vi "运维调试_氨氮.vi"() -> ()   [LabVIEW 2016, in "斯坦道氨氮.lvlib"]
uses:
  <vilib>/Utility/miscctls.llb/LVPointTypeDef.ctl
  <vilib>/Utility/config.llb/NI_LVConfig.lvlib
  <vilib>/ptbypt/NI_PtbyPt.lvlib
panel:
  in  "定时设置":cluster{"启动":bool, "控制命令":T1}(xcontrol)
  out "二级权限":bool
  out "一级权限":bool
  out "输入密码":u32
  out "布尔":bool
  in  "仪器参数设置":bool
  in  "流程固件":bool
  in  "量程参数读取":T2
  in  "模块启用":bool
  in  "串口设置":bool
  in  "公式一键写入":bool
  in  "流程路径":path=path "C:/Users/STD/Documents/斯坦道流程文件/流程.xml"
  in  "曲线模型":cluster{"X^2":dbl, "X":dbl, "B":dbl}(xcontrol)
  out "字符串":string
  in  "质控参数设置":bool
  in  "自动测试量程配置":T3
  out "温度2":sgl
  out "温度1":sgl
  out "ADC":sgl
  out "固件版本号":string
  in  "数组":string[](array[string])
  in  "量程切换阈值写入":bool
  in  "量程切换阈值读取":bool
  in  "参数下拉列表":enum16{"总磷", "总氮", "氨氮"}(ring)=enum."氨氮"
  in  "量程下拉列表":enum16{"低量程", "高量程"}(ring)
  in  "测量模式下拉列表":enum16{"水样测量", "零点核查", "跨度核查", "标样核查", "加标回收"}(ring)
  in  "公式":cluster{"X^2":dbl, "X":dbl, "b":dbl}
  in  "写公式":bool
  in  "读公式":bool
  in  "返回":bool
  in  "设置":bool
  out "序列号":string="序列号"
  out "测量数据":T4(xcontrol)
  out "集成报警信息":string
  out "总磷总氮运行状态":T5(xcontrol)
  in  "停止":bool
  in  "手动启动":bool
  in  "单步测试":bool
  in  "总磷氨氮调试":u16[](xcontrol)
  out "F3":sgl format="%#.6f"
  out "F2":sgl format="%#.6f"
  out "F1":sgl format="%#.6f"
  out "F0":sgl format="%#.6f"
  out "多列列表框":i32(listbox)
  # "参数设置"
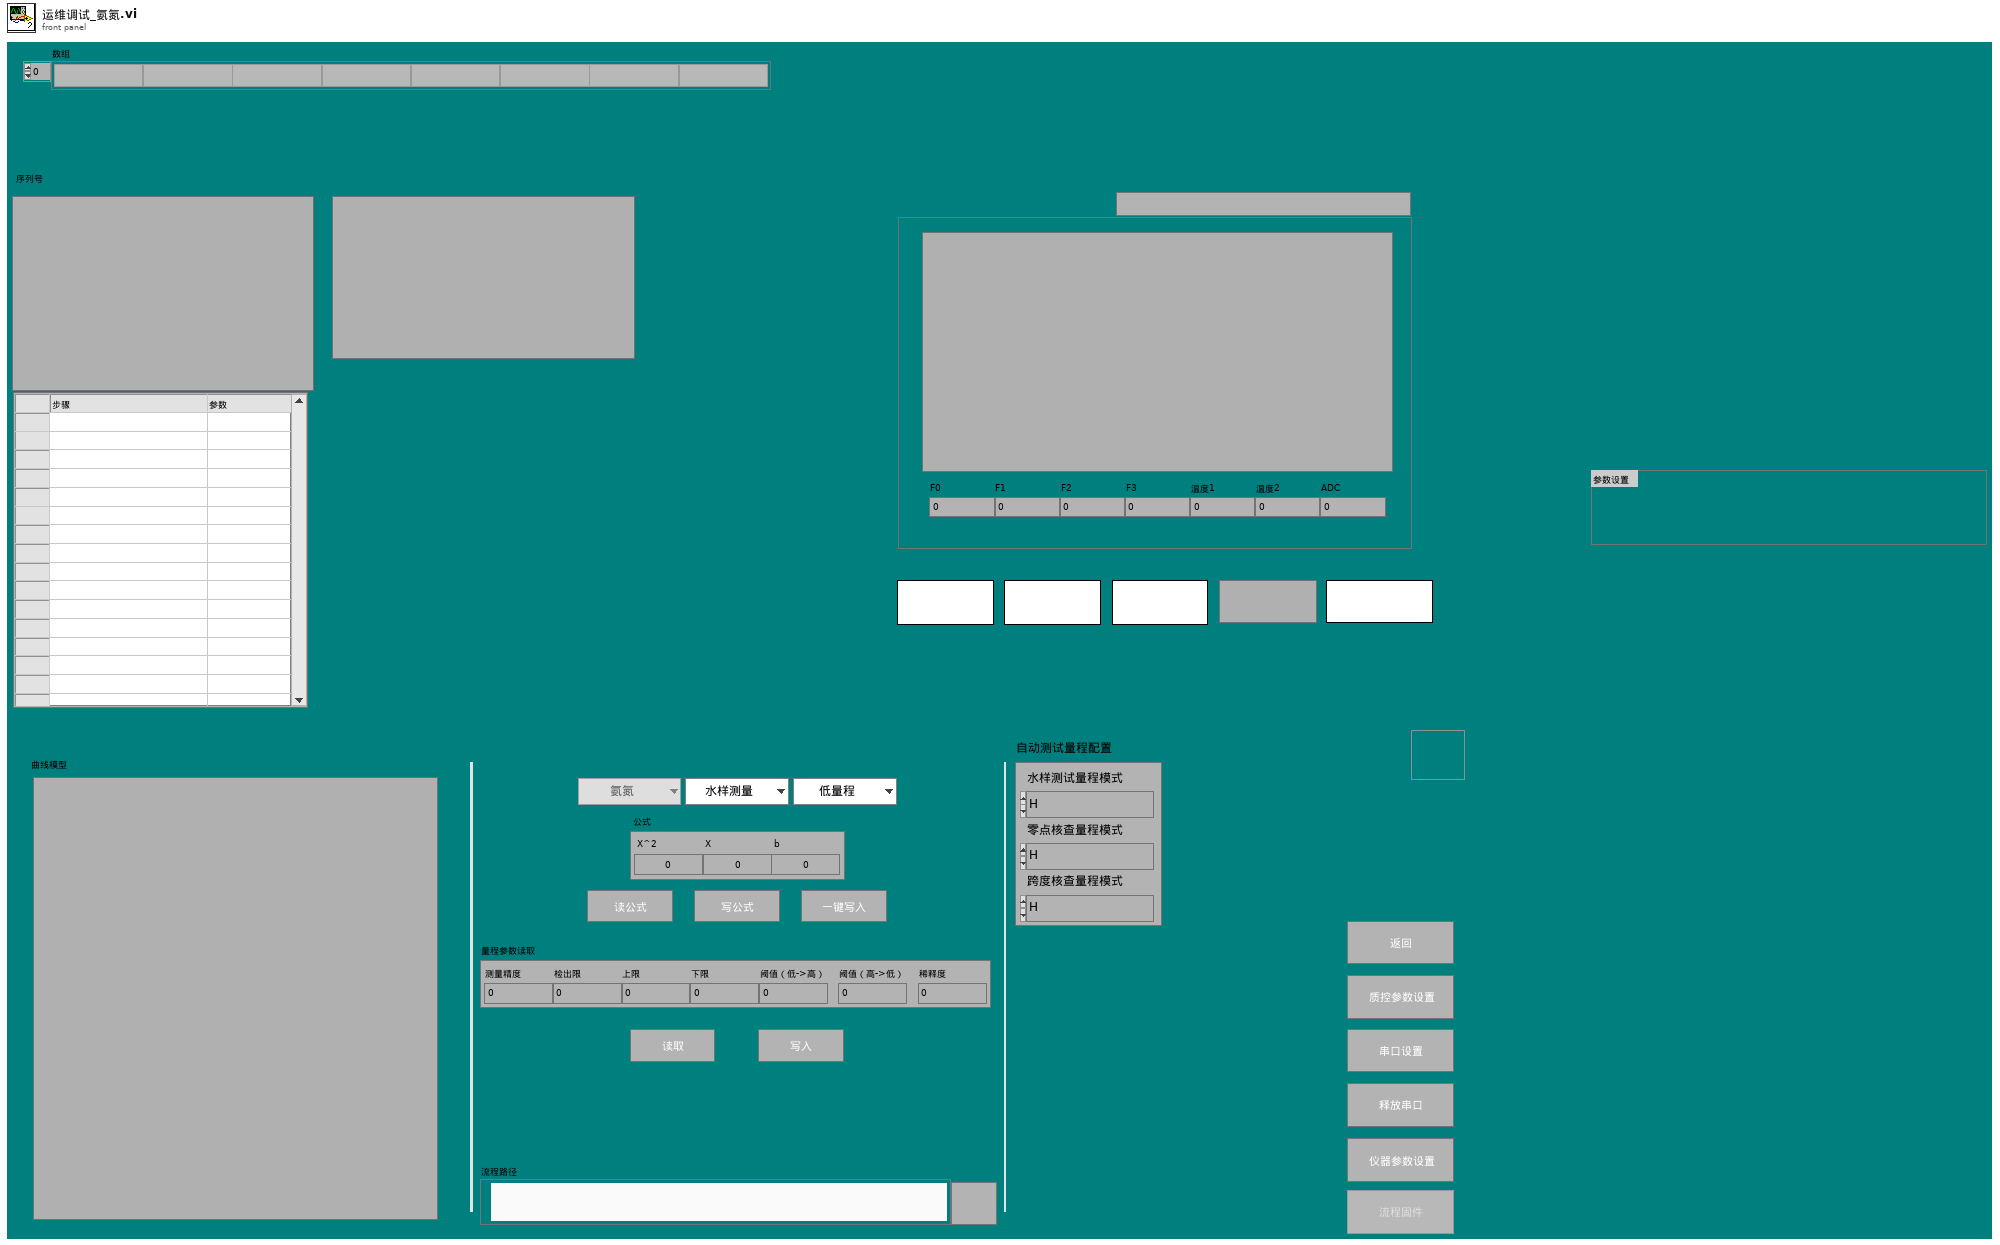
[diagram p1: front panel]
types:
  T1 = typedef "定时设置.xctl/国标控制命令.ctl" = enum16{"启动测量", "标样核查", "零点核查", "跨度核查", "空白测试", "平行样测试", "加标回收", "空白校准", "标样校准", "初始化（清洗）", "停止测试", "仪器重启", "校时", "模式设置", "测量间隔设置"}
  T2 = cluster{"测量精度":dbl, "检出限":dbl, "上限":dbl, "下限":dbl, "阈值（低->高）":dbl, "阈值（高->低）":dbl, "稀释度":dbl}
  T3 = cluster{"水样测试量程模式":enum16{"H", "L", "AUTO"}, "空白核查量程模式":enum16{"H", "L", "AUTO"}, "跨度核查量程模式":enum16{"H", "L", "AUTO"}}
  T4 = cluster{"flowid":u16, "测量精度":u16, "测量数据区":cluster{"因子编码":u32, "单位":u16, "标样参考值":sgl, "水样数据时间":timestamp, "水样实测值":sgl, "水样数据标识":string, "标样数据时间":timestamp, "标样实测值":sgl, "标样数据标识":string, "空白数据时间":timestamp, "空白实测值":sgl, "空白数据标识":string, "零点核查数据时间":timestamp, "零点核查实测值":sgl, "零点核查数据标识":string, "跨度核查数据时间":timestamp, "跨度核查实测值":sgl, "跨度核查数据标识":string, "加标回收数据时间":timestamp, "加标回收实测值":sgl, "加标回收数据标识":string, "平行样数据时间":timestamp, "平行样实测值":sgl, "平行样数据标识":string, "F0":sgl, "F1":sgl, "F2":sgl, "F3":sgl, "F4":sgl, "F5":sgl, "F6":sgl, "F7":sgl, "温度":sgl, "湿度":sgl, "X值":sgl, "fidrange":sgl}}
  T5 = cluster{"系统时间":timestamp, "工作状态":enum16{"空闲", "水样测试", "标样核查", "零点核查", "跨度核查", "空白测试", "平行样测试", "加标回收", "空白校准", "标样校准", "初始化（清洗）"}, "测量模式":enum16{"待机", "连续模式", "周期模式", "定点模式", "受控模式", "手动模式"}, "告警代码":u16, "故障代码":u16, "日志代码":u16, "软件版本":u16, "F0":sgl, "F1":sgl, "F2":sgl, "F3":sgl, "T":sgl, "H":sgl, "id":u16, "flowid":u16, "量程":u16, "总磷控温温度1":sgl, "营养盐控温温度2":sgl, "ADC":sgl}
  T6 = typedef "NI_LVConfig.lvlib/Config Data RefNum.ctl" = refnum<k1>
  T7 = typedef "LVPointTypeDef.ctl" = cluster{"Horizontal":i16, "Vertical":i16}
  T8 = cluster{"因子编码":u32, "单位":u16, "标样参考值":sgl, "水样数据时间":timestamp, "水样实测值":sgl, "水样数据标识":string, "标样数据时间":timestamp, "标样实测值":sgl, "标样数据标识":string, "空白数据时间":timestamp, "空白实测值":sgl, "空白数据标识":string, "零点核查数据时间":timestamp, "零点核查实测值":sgl, "零点核查数据标识":string, "跨度核查数据时间":timestamp, "跨度核查实测值":sgl, "跨度核查数据标识":string, "加标回收数据时间":timestamp, "加标回收实测值":sgl, "加标回收数据标识":string, "平行样数据时间":timestamp, "平行样实测值":sgl, "平行样数据标识":string, "F0":sgl, "F1":sgl, "F2":sgl, "F3":sgl, "F4":sgl, "F5":sgl, "F6":sgl, "F7":sgl, "温度":sgl, "湿度":sgl, "X值":sgl, "fidrange":u16}
  T9 = enum16{"空闲", "水样测试", "标样核查", "零点核查", "跨度核查", "空白测试", "平行样测试", "加标回收", "空白校准", "标样校准", "初始化（清洗）"}
  T10 = enum32{"Bad", "Idle", "Run top level", "Running"}
  T11 = typedef "定时设置.xctl/周期模式设置.ctl" = enum16{"不启用", "定点模式", "间隔模式"}
  T12 = typedef "定时设置.xctl/定点周期设置.ctl" = cluster{"启动命令":T13, "启动命令 2":T13, "启动命令 3":T13, "启动命令 4":T13, "启动命令 5":T13, "启动命令 6":T13, "启动命令 7":T13, "启动命令 8":T13, "启动命令 9":T13, "启动命令 10":T13, "启动命令 11":T13, "启动命令 12":T13, "启动命令 13":T13, "启动命令 14":T13, "启动命令 15":T13, "启动命令 16":T13, "启动命令 17":T13, "启动命令 18":T13, "启动命令 19":T13, "启动命令 20":T13, "启动命令 21":T13, "启动命令 22":T13, "启动命令 23":T13, "启动命令 24":T13}
  T13 = typedef "定时设置.xctl/启动命令选择.ctl" = u16
  T14 = typedef "定时设置.xctl/间隔启动设置.ctl" = cluster{"启动命令":T13, "启动间隔":dbl, "启动次数":i32}
  T15 = enum8{"Enabled", "Disabled", "Disabled and Grayed Out"}
  T16 = cluster{"启动模式":enum16{"跨度核查", "水样测量", "空白核查", "标样核查", "加标回收"}, "启动参数":u16, "量程":enum16{"低量程", "高量程"}}
  T17 = cluster{"时间标识":timestamp, "设备":string, "日志信息":string, "流程参数":string}
  T18 = cluster{"时间标识":timestamp, "设备":string, "日志信息":string}
  T19 = typedef "LVRowAndColumnUnsignedTypeDef.ctl" = cluster{"Row":u32, "Column":u32}
  T20 = cluster{"参数下拉列表":enum16{"总磷", "总氮", "氨氮"}, "测量模式下拉列表":enum16{"水样测量", "零点核查", "跨度核查", "标样核查", "加标回收"}, "量程下拉列表":enum16{"低量程", "高量程"}}
  T21 = cluster{"站号":u16, "量程切换":enum32{"H", "L", "AUTO"}, "控制命令":enum16{"启动测量", "标样核查", "零点核查", "跨度核查", "空白测试", "平行样测试", "加标回收", "空白校准", "标样校准", "初始化（清洗）", "停止测试", "仪器重启", "校时", "模式设置", "测量间隔设置"}, "模式设置":enum16{"待机", "连续模式", "周期模式", "定点模式", "受控模式", "手动模式"}, "测量间隔":u16}
  T22 = cluster{"跨度值":dbl, "零点标准液浓度":dbl, "跨度标准液浓度":dbl, "标准液标准浓度":dbl}
  T23 = cluster{"确定":bool, "跨度值":dbl, "零点标准液浓度":dbl, "跨度标准液浓度":dbl, "标准液标准浓度":dbl}
  T24 = cluster{"测量量程":dbl, "测量精度":dbl, "测量间隔":dbl, "消解温度":dbl, "消解时长":dbl, "空白校准时间":timestamp, "曲线截距":dbl, "曲线斜率":dbl, "测量检出限":dbl, "测量信号值":dbl, "线性相关系数":dbl, "二次多项式系数":dbl, "标样校准时间":timestamp, "单位":u16}
  T25 = cluster{"确定":bool, "测量量程":dbl, "测量精度":dbl, "测量间隔":dbl, "消解温度":dbl, "消解时长":dbl, "空白校准时间":timestamp, "曲线截距":dbl, "曲线斜率":dbl, "测量检出限":dbl, "测量信号值":dbl, "线性相关系数":dbl, "二次多项式系数":dbl, "标样校准时间":timestamp, "单位":u16}
  T26 = cluster{"测量精度":u16, "检出限":dbl, "上限":dbl, "下限":dbl, "阈值（低->高）":dbl, "阈值（高->低）":dbl, "稀释度":dbl}
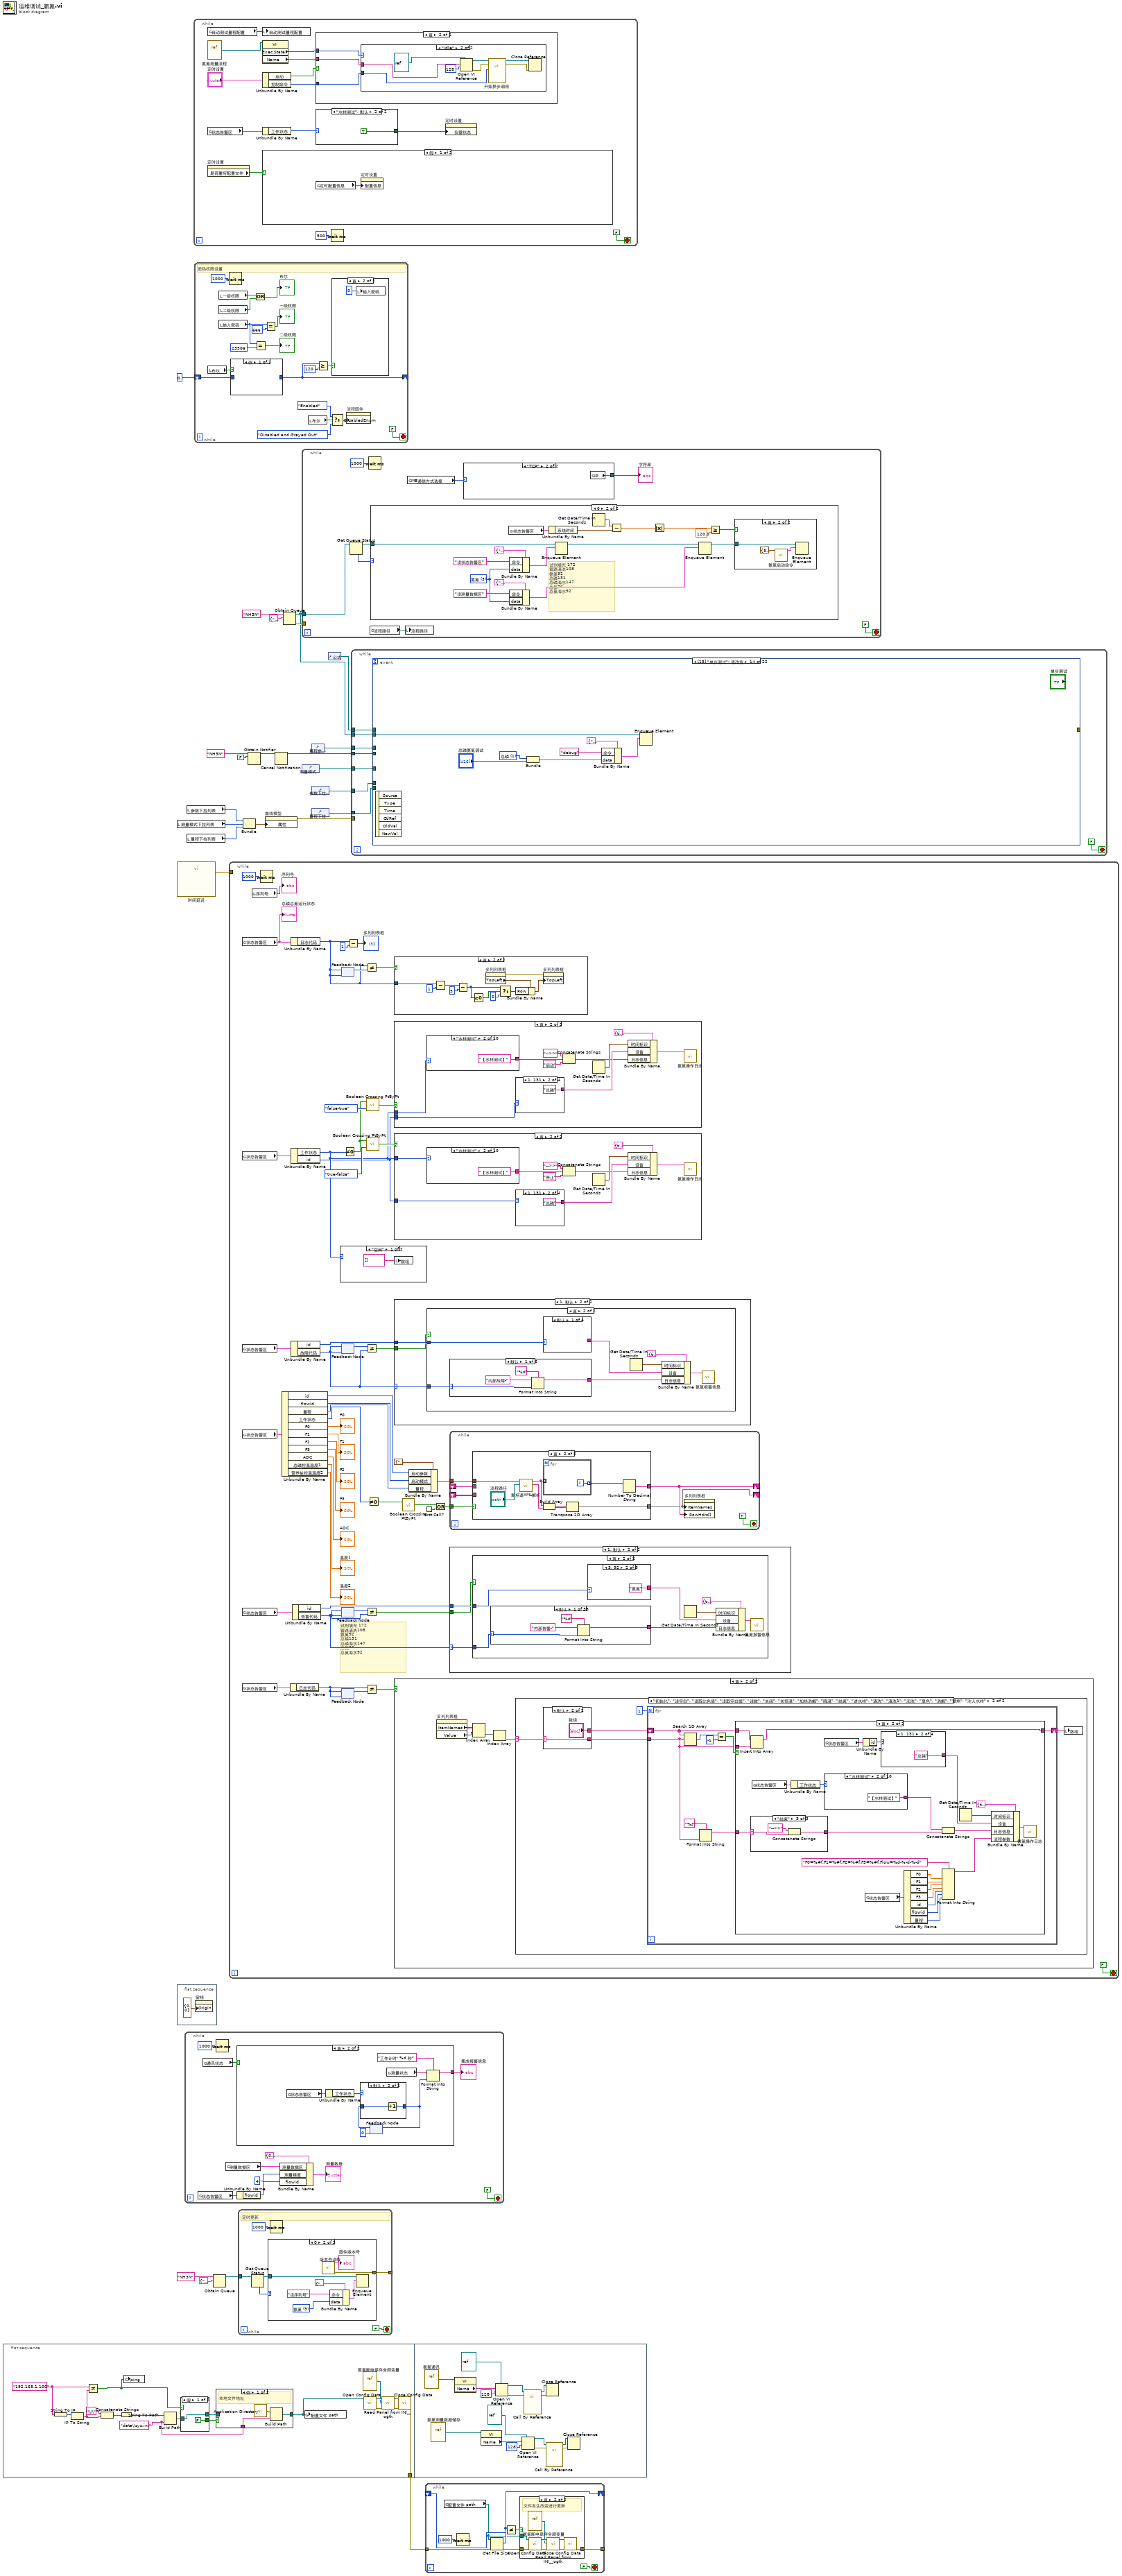
[diagram p0: block diagram]
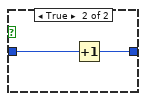
[diagram p4: hidden frame]
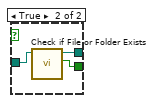
[diagram p5: hidden frame]
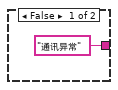
[diagram p8: hidden frame]
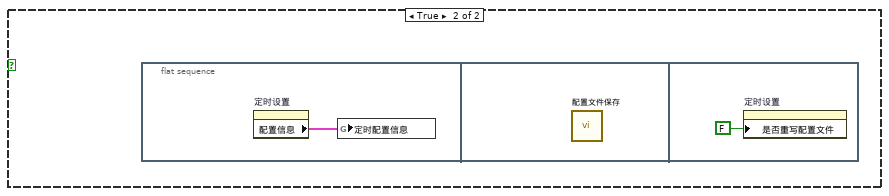
[diagram p10: hidden frame]
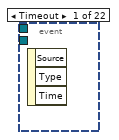
[diagram p14: hidden frame]
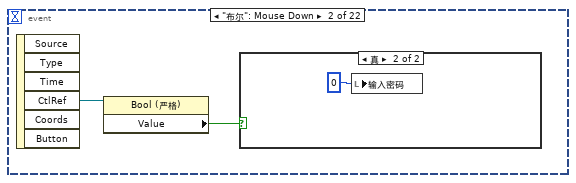
[diagram p15: hidden frame]
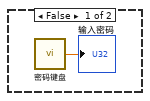
[diagram p16: hidden frame]
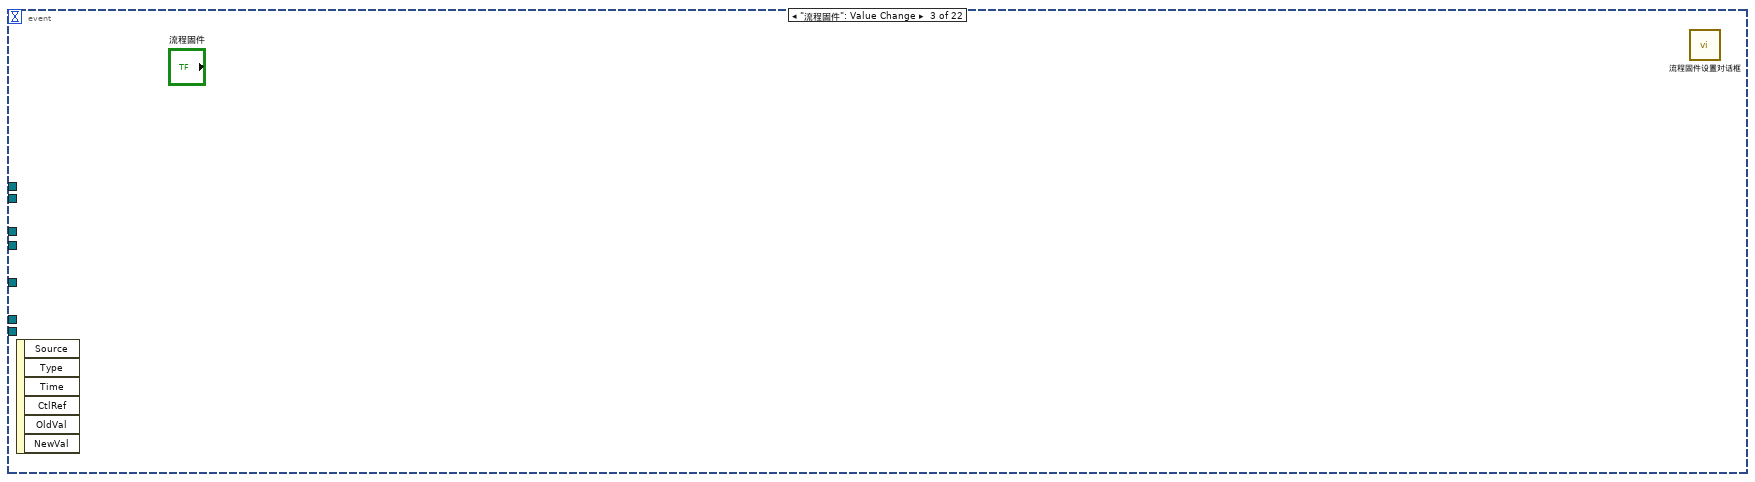
[diagram p17: hidden frame]
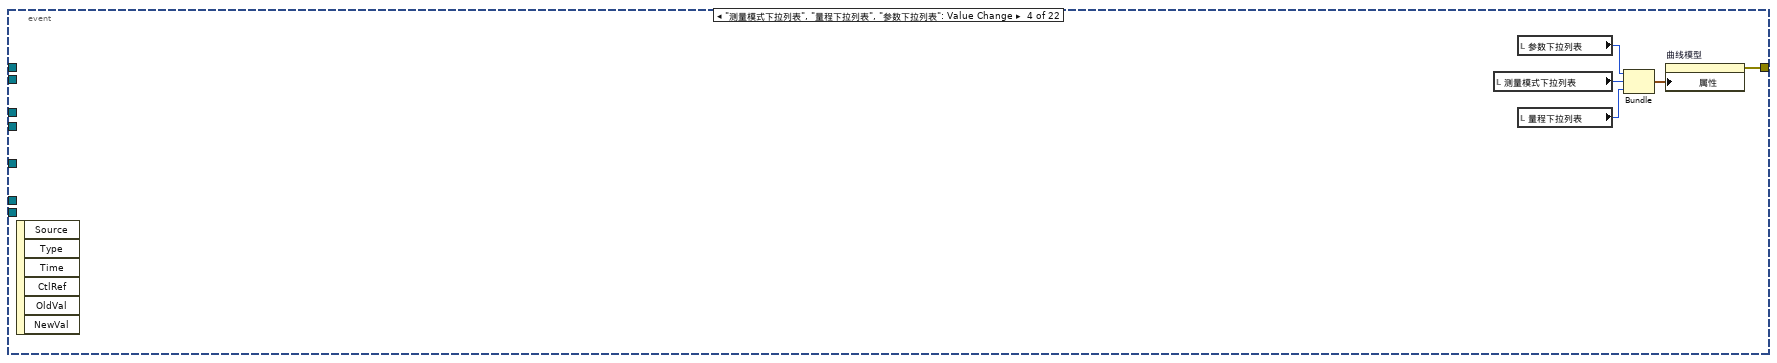
[diagram p18: hidden frame]
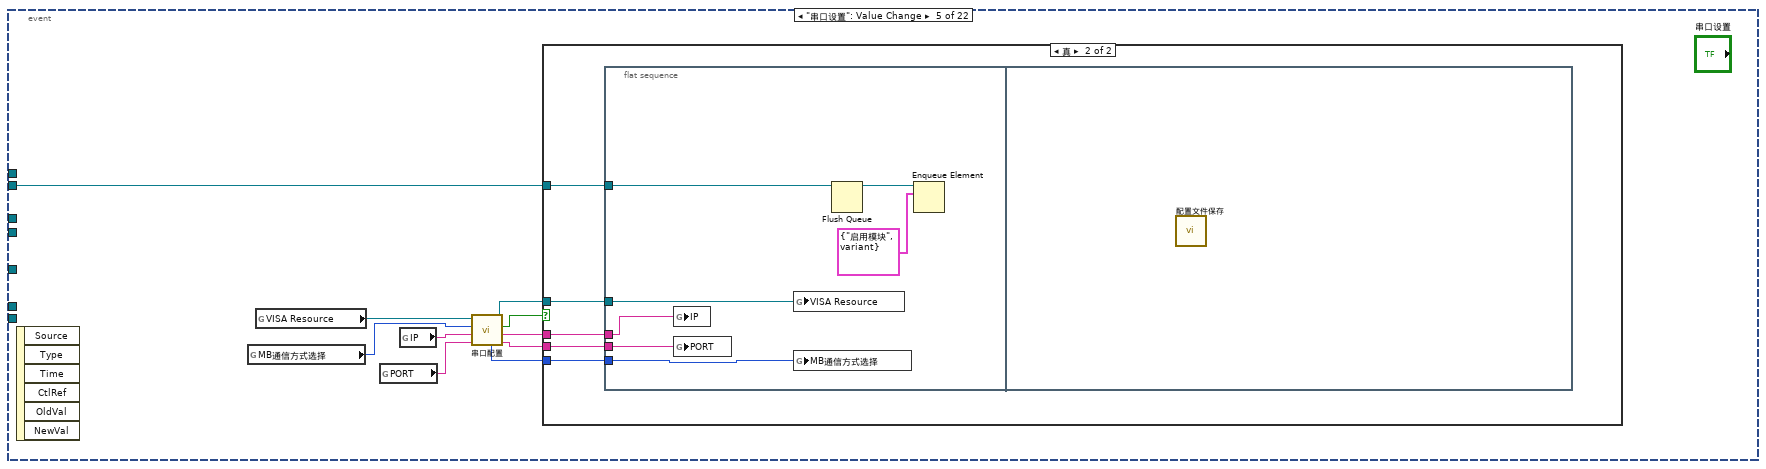
[diagram p19: hidden frame]
diagram:
  n1 = flat-sequence {
    tunnel: [w25] -> w1
    frame #0 {
      w36 = "data\\sys.ini" ("名称或相对路径")
      w28 = "192.168.1.100" ("名称")
      n2 = String To IP(1:w28) -> (0:w35:u32)
      n3 = IP To String(2:w35) -> (0:w32:string)  [unwired: 1 in]
      n4 = Not Equal?(x=w28, y=w32) -> (x != y?=w37:bool)
      n5 = Concatenate Strings("\\\\" ("字符串"), w32) -> (w33:string)
      n6 = String To Path(string=w33) -> (path=w27:path)
      n7 = global write "VAR氨氮全局变量.vi" "ping"(w37) -> ()
      n8 = Build Path(base path=w27, name or relative path=w36) -> (appended path=w31:path)
      n9 = case shown="假" w37 {
        tunnel: w31 -> [w43 w47]
        tunnel: [w43 w46] -> w30
        tunnel: [FALSE w45] -> w29
        frame False {
        }
        frame True {
          n10 = call <vilib>:"Check if File or Folder Exists.vi"("path"=w47) -> ("file or folder exists?"=w45:bool, "dup path"=w46:path)  [unwired: 8 in, 1 out]
        }
      }
      n11 = case shown="假" w29 {
        tunnel: w30 -> [_ w51]
        tunnel: [w49 w51] -> w26
        tunnel: w36 -> [w48 _]
        frame False {
          # "本地文件地址"
          n12 = call <vilib>:"Application Directory.vi"() -> ("Application Directory"=w50:path)
          n13 = Build Path(base path=w50, name or relative path=w48) -> (appended path=w49:path)
        }
        frame True {
          # "网络共享地址"
        }
      }
      n14 = global write "VAR氨氮全局变量.vi" "配置文件 path"(w26) -> ()
      n15 = vi-ref "氨氮断电保存全局变量.vi"() -> (w41:refnum<vi>)
      n16 = call <vilib>:"Open Config Data.vi"("configuration file path"=w26) -> ("error out"=w39:errorcluster, "refnum"=w42:T6)  [unwired: 8 in, 1 out]
      n17 = call <userlib>:"Read Panel from INI__ogtk.vi"("error in (no error)"=w39, "VI ref"=w41, "refnum"=w42) -> ("error out"=w38:errorcluster, "refnum out"=w40:T6)  [unwired: 7 in]
      n18 = call <vilib>:"Close Config Data.vi"("error in (no error)"=w38, "refnum"=w40) -> ("error out"=w25:errorcluster)  [unwired: 8 in, 1 out]
    }
    frame #1 {
      n19 = vi-ref "氨氮通讯.vi"() -> (w67:refnum<vi>)
      n20 = vi-ref "氨氮测量数据储存.vi"() -> (w59:refnum<vi>)
      n21 = property class="VI"(reference=w67) -> ("Name"=w66:string)  [unwired: 1 in, 2 out]
      n22 = property class="VI"(reference=w59) -> ("Name"=w52:string)  [unwired: 1 in, 2 out]
      n23 = Open VI Reference(type specifier VI Refnum (for type only)=refnum<vi> refnum, vi path=w66, options=128 ("选项")) -> (vi reference=w64:refnum<vi>, error out=w62:errorcluster)  [unwired: 3 in]
      n24 = Open VI Reference(type specifier VI Refnum (for type only)=refnum<vi> refnum, vi path=w52, options=128 ("选项")) -> (vi reference=w54:refnum<vi>, error out=w56:errorcluster)  [unwired: 3 in]
      n25 = call-by-ref "?"(reference=w64, error in=w62) -> (reference out=w60:refnum<vi>, error out=w61:errorcluster)  [unwired: 12 in]
      n26 = Close Reference(reference=w60, error in (no error)=w61) -> ()  [unwired: 1 out]
      n27 = call-by-ref "?"(reference=w54, error in=w56) -> (reference out=w58:refnum<vi>, error out=w57:errorcluster)  [unwired: 12 in]
      n28 = Close Reference(reference=w58, error in (no error)=w57) -> ()  [unwired: 1 out]
    }
  }
  n29 = local read "测量模式下拉列表"() -> (w4:enum16{"水样测量", "零点核查", "跨度核查", "标样核查", "加标回收"})
  n30 = call "时间延迟"() -> ("error out"=w16:errorcluster)  [unwired: 11 in]
  n31 = flat-sequence {
    frame #0 {
      n32 = property on="窗格" class="Pane"("Origin"=T7 {"Horizontal"=0, "Vertical"=0} ("原点")) -> ()  [unwired: 2 in, 2 out]
    }
  }
  n33 = while {
    stop <- FALSE stop-if-true
    n34 = global read "VAR氨氮全局变量.vi" "状态告警区"() -> (w74:T5)
    n35 = global read "VAR氨氮全局变量.vi" "通讯状态"() -> (w76:bool)
    n36 = Wait (ms)(milliseconds to wait=u32 1000 ("等待时间（毫秒）")) -> ()  [unwired: 1 out]
    n37 = global read "VAR氨氮全局变量.vi" "测量数据区"() -> (w71:T8)
    n38 = case shown="真" w76 {
      tunnel: ["通讯异常" ("集成报警信息") w81] -> w75
      frame False {
      }
      frame True {
        n39 = global read "VAR氨氮全局变量.vi" "状态告警区"() -> (w87:T5)
        n40 = Unbundle By Name(w87) -> ("工作状态"=w86:T9)
        n41 = feedback #1(0) -> (w84:i32)
        n42 = case shown="默认" w86 {
          tunnel: w84 -> [_ w89]
          tunnel: [_ w88] -> w82
          frame "空闲" {
          }
          frame Default {
            n43 = Increment(x=w89) -> (x+1=w88:i32)
          }
        }
        n44 = feedback-in #1(w82) -> ()
        n45 = global read "VAR氨氮全局变量.vi" "测量状态"() -> (w80:string)
        n46 = Format Into String(format string="工作计时: %d 秒" ("格式字符串"), initial string=w80, w82) -> (resulting string=w81:string)  [unwired: 1 in, 1 out]
      }
    }
    "集成报警信息" <- w75
    n47 = Unbundle By Name(w74) -> ("flowid"=w73:u16)
    n48 = Bundle By Name(cluster=T4 {"flowid"=0, "测量精度"=0, "测量数据区"={"因子编码"=0, "单位"=0, "标样参考值"=0.0, "水样数据时间"=timestamp(0 s since 1904-01-01), "水样实测值"=0.0, "水样数据标识"="", "标样数据时间"=timestamp(0 s since 1904-01-01), "标样实测值"=0.0, "标样数据标识"="", "空白数据时间"=timestamp(0 s since 1904-01-01), "空白实测值"=0.0, "空白数据标识"="", "零点核查数据时间"=timestamp(0 s since 1904-01-01), "零点核查实测值"=0.0, "零点核查数据标识"="", "跨度核查数据时间"=timestamp(0 s since 1904-01-01), "跨度核查实测值"=0.0, "跨度核查数据标识"="", "加标回收数据时间"=timestamp(0 s since 1904-01-01), "加标回收实测值"=0.0, "加标回收数据标识"="", "平行样数据时间"=timestamp(0 s since 1904-01-01), "平行样实测值"=0.0, "平行样数据标识"="", "F0"=0.0, "F1"=0.0, "F2"=0.0, "F3"=0.0, "F4"=0.0, "F5"=0.0, "F6"=0.0, "F7"=0.0, "温度"=0.0, "湿度"=0.0, "X值"=0.0, "fidrange"=0.0}} ("测量数据"), "测量数据区"=w71, "测量精度"=u16 4, "flowid"=w73) -> (→"测量数据":T4)
  }
  n49 = local read "参数下拉列表"() -> (w5:enum16{"总磷", "总氮", "氨氮"})
  n50 = local read "量程下拉列表"() -> (w3:enum16{"低量程", "高量程"})
  n51 = while {
    stop <- FALSE stop-if-true
    n52 = global read "氨氮断电保存全局变量.vi" "自动测试量程配置"() -> (w100:T3)
    n53 = vi-ref "氨氮测量流程.vi"() -> (w99:refnum<vi>)
    n54 = global read "VAR氨氮全局变量.vi" "状态告警区"() -> (w93:T5)
    n55 = property on="定时设置" class="定时设置 (严格)"() -> ("是否重写配置文件"=w90:bool)  [unwired: 2 in, 2 out]
    n56 = local write "自动测试量程配置"(w100) -> ()
    n57 = property class="VI"(reference=w99) -> ("Exec.State"=w97:T10, "Name"=w98:string)  [unwired: 1 in, 2 out]
    n58 = Unbundle By Name("定时设置") -> ("启动"=w94:bool, "控制命令"=w95:T1)
    n59 = Unbundle By Name(w93) -> ("工作状态"=w92:T9)
    n60 = case shown="假" w90 {
      frame False {
        n61 = global read "氨氮断电保存全局变量.vi" "定时配置信息"() -> (w103:cluster{"周期模式":T11, "定点周期":T12, "间隔启动":T14})
        n62 = property on="定时设置" class="定时设置 (严格)"("配置信息"=w103) -> ()  [unwired: 2 in, 2 out]
      }
      frame True {
        n63 = flat-sequence {
          frame #0 {
            n64 = property on="定时设置" class="定时设置 (严格)"() -> ("配置信息"=w104:cluster{"周期模式":T11, "定点周期":T12, "间隔启动":T14})  [unwired: 2 in, 2 out]
            n65 = global write "氨氮断电保存全局变量.vi" "定时配置信息"(w104) -> ()
          }
          frame #1 {
            n66 = call "配置文件保存.vi"() -> ()  [unwired: 12 in]
          }
          frame #2 {
            n67 = property on="定时设置" class="定时设置 (严格)"("是否重写配置文件"=FALSE) -> ()  [unwired: 2 in, 2 out]
          }
        }
      }
    }
    n68 = case shown="真" w94 {
      tunnel: w98 -> [_ w109]
      tunnel: w95 -> [_ w108]
      tunnel: w97 -> [_ w107]
      frame False {
      }
      frame True {
        n69 = case shown="\"Idle\"" w107 {
          tunnel: w109 -> [_ w113]
          tunnel: w108 -> [_ w111]
          frame "Bad", Default {
          }
          frame "Idle" {
            n70 = Open VI Reference(type specifier VI Refnum (for type only)=refnum<vi> refnum, vi path=w113, options=128 ("选项")) -> (vi reference=w114:refnum<vi>, error out=w115:errorcluster)  [unwired: 3 in]
            n71 = call-by-ref "开始异步调用"(reference=w114, error in=w115, "控制命令"=w111) -> (reference out=w116:refnum<vi>, error out=w117:errorcluster)  [unwired: 11 in]
            n72 = Close Reference(reference=w116, error in (no error)=w117) -> ()  [unwired: 1 out]
          }
        }
      }
    }
    n73 = case shown="\"水样测试\", 默认" w92 {
      tunnel: [_ TRUE] -> w91
      frame "空闲" {
      }
      frame "水样测试", Default {
      }
    }
    n74 = Wait (ms)(milliseconds to wait=u32 500 ("等待时间（毫秒）")) -> ()  [unwired: 1 out]
    n75 = property on="定时设置" class="定时设置 (严格)"("仪器状态"=w91) -> ()  [unwired: 2 in, 2 out]
  }
  n76 = while {
    shift-right: [w120] -> _
    shift-left: u32 0 ("等待时间（毫秒）") -> [w121]
    stop <- FALSE stop-if-true
    # "密码权限设置"
    n77 = local read "布尔"() -> (w122:bool)
    n78 = local read "一级权限"() -> (w129:bool)
    n79 = local read "二级权限"() -> (w130:bool)
    n80 = local read "输入密码"() -> (w133:u32)
    n81 = Wait (ms)(milliseconds to wait=u32 1000 ("等待时间（毫秒）")) -> ()  [unwired: 1 out]
    n82 = case shown="假" w122 {
      tunnel: w121 -> [_ w139]
      tunnel: [_ w138] -> w120
      frame False {
      }
      frame True {
        n83 = Increment(x=w139) -> (x+1=w138:u32)
      }
    }
    n84 = Or(x=w129, y=w130) -> (x .or. y?=→"布尔":bool)
    n85 = Equal?(x=w133, y=u32 23506) -> (x = y?=→"二级权限":bool)
    n86 = Equal?(x=w133, y=u32 666) -> (x = y?=→"一级权限":bool)
    n87 = local read "布尔"() -> (w124:bool)
    n88 = Greater Or Equal?(x=w120, y=u32 120) -> (x >= y?=w118:bool)
    n89 = Select(t=T15."Enabled" ("禁用"), s=w124, f=T15."Disabled and Grayed Out") -> (s? t:f=w125:T15)
    n90 = case shown="真" w118 {
      frame False {
      }
      frame True {
        n91 = local write "输入密码"(u32 0 ("输入密码")) -> ()
      }
    }
    n92 = property on="流程固件" class="Bool"("DisabledEnum"=w125) -> ()  [unwired: 2 in, 2 out]
  }
  n93 = Obtain Queue(name (unnamed)="NH3N" ("名称（未命名）"), element data type=cluster{"命令":string, "data":variant} {"命令"="", "data"=variant}) -> (queue out=w13:refnum<queue>)  [unwired: 3 in, 2 out]
  n94 = while {
    tunnel: w16 -> [_]
    stop <- FALSE stop-if-true
    # "试剂填充 172 \n管路清洗108\n氨氮92\n总磷131\n总磷海水147\n总氮76\n总氮海水92"
    n95 = global read "VAR氨氮全局变量.vi" "状态告警区"() -> (w173:T5)
    "总磷总氮运行状态" <- w173
    n96 = global read "VAR氨氮全局变量.vi" "状态告警区"() -> (w160:T5)
    n97 = global read "VAR氨氮全局变量.vi" "状态告警区"() -> (w165:T5)
    n98 = global read "VAR氨氮全局变量.vi" "状态告警区"() -> (w181:T5)
    n99 = global read "VAR氨氮全局变量.vi" "状态告警区"() -> (w170:T5)
    n100 = global read "VAR氨氮全局变量.vi" "状态告警区"() -> (w158:T5)
    n101 = global read "VAR氨氮全局变量.vi" "序列号"() -> (→"序列号":string)
    n102 = Wait (ms)(milliseconds to wait=u32 1000 ("等待时间（毫秒）")) -> ()  [unwired: 1 out]
    n103 = Unbundle By Name(w181) -> ("id"=w178:u16, "flowid"=w180:u16, "量程"=w179:u16, "工作状态"=w148:T9, "F0"=→"F0":sgl, "F1"=→"F1":sgl, "F2"=→"F2":sgl, "F3"=→"F3":sgl, "ADC"=→"ADC":sgl, "总磷控温温度1"=→"温度1":sgl, "营养盐控温温度2"=→"温度2":sgl)
    n104 = Unbundle By Name(w158) -> ("日志代码"=w157:u16)
    n105 = Unbundle By Name(w173) -> ("日志代码"=w154:u16)
    n106 = Unbundle By Name(w160) -> ("工作状态"=w141:T9, "id"=w140:u16)
    n107 = Unbundle By Name(w165) -> ("id"=w164:u16, "故障代码"=w161:u16)
    n108 = Unbundle By Name(w170) -> ("id"=w169:u16, "告警代码"=w166:u16)
    n109 = case shown="\"空闲\"" w141 {
      frame "空闲" {
        n110 = local write "数组"(string[] [] ("数组")) -> ()
      }
      frame "水样测试", Default {
      }
    }
    n111 = feedback-in #2(w154) -> ()
    n112 = feedback #2(w154) -> (w186:u16)
    n113 = feedback #3(w161) -> (w162:u16)
    n114 = feedback-in #3(w161) -> ()
    n115 = feedback #4(w166) -> (w167:u16)
    n116 = feedback-in #4(w166) -> ()
    n117 = feedback #5(w157) -> (w159:u16)
    n118 = feedback-in #5(w157) -> ()
    n119 = Not Equal To 0?(x=w141) -> (x != 0?=w143:bool)
    n120 = Subtract(x=w154, y=1) -> (x-y=→"多列列表框":i32)
    n121 = Not Equal?(x=w154, y=w186) -> (x != y?=w185:bool)
    n122 = Not Equal?(x=w162, y=w161) -> (x != y?=w163:bool)
    n123 = Not Equal?(x=w167, y=w166) -> (x != y?=w168:bool)
    n124 = Not Equal?(x=w157, y=w159) -> (x != y?=w156:bool)
    n125 = call <vilib>:"Boolean Crossing PtByPt.vi"("direction"=enum16{"either", "false-true", "true-false"}."false-true", "input"=w143) -> ("crossing"=w145:bool)  [unwired: 1 in]
    n126 = call <vilib>:"Boolean Crossing PtByPt.vi"("direction"=enum16{"either", "false-true", "true-false"}."true-false", "input"=w143) -> ("crossing"=w142:bool)  [unwired: 1 in]
    n127 = Not Equal To 0?(x=w148) -> (x != 0?=w183:bool)
    n128 = case shown="真" w185 {
      tunnel: w154 -> [_ w396]
      frame False {
      }
      frame True {
        n129 = Subtract(x=w396, y=1) -> (x-y=w394:i32)
        n130 = Subtract(x=w394, y=5) -> (x-y=w398:i32)
        n131 = Greater Or Equal To 0?(x=w398) -> (x >= 0?=w397:bool)
        n132 = property on="多列列表框" class="MCListbox (严格)"() -> (error out=w402:errorcluster, "TopLeft"=w403:T19)  [unwired: 2 in, 1 out]
        n133 = Select(t=w398, s=w397, f=0) -> (s? t:f=w399:i32)
        n134 = Bundle By Name(cluster=w403, "Row"=w399) -> (w404:T19)
        n135 = property on="多列列表框" class="MCListbox (严格)"(error in=w402, "TopLeft"=w404) -> ()  [unwired: 1 in, 2 out]
      }
    }
    n136 = case shown="真" w145 {
      tunnel: w140 -> [_ w216]
      tunnel: w141 -> [_ w215]
      frame False {
      }
      frame True {
        n137 = case shown="\"水样测试\"" w215 {
          tunnel: [_ "【水样测试】" ("字符串") "【标样核查】" ("字符串") "【零点核查】" ("字符串") "【跨度核查】" ("字符串") "【空白测试】" ("字符串") "【平行样测试】" ("字符串") "【加标回收】" ("字符串") "【空白校准】" ("字符串") "【标样校准】" ("字符串")] -> w214
          frame "空闲", Default {
          }
          frame "水样测试" {
          }
          frame "标样核查" {
          }
          frame "零点核查" {
          }
          frame "跨度核查" {
          }
          frame "空白测试" {
          }
          frame "平行样测试" {
          }
          frame "加标回收" {
          }
          frame "空白校准" {
          }
          frame "标样校准" {
          }
        }
        n138 = case shown="1, 131" w216 {
          tunnel: [_ "总磷" ("table输入") "氨氮" ("table输入") "总氮" ("table输入")] -> w218
          frame Default {
          }
          frame 1, 131 {
          }
          frame 3, 92 {
          }
          frame 2, 76 {
          }
        }
        n139 = Concatenate Strings("-->>" ("字符串"), w214, "启动" ("字符串")) -> (w213:string)
        n140 = Get Date/Time In Seconds() -> (seconds since 1Jan1904=w219:timestamp)
        n141 = Bundle By Name(cluster=T17 {"时间标识"=timestamp(0 s since 1904-01-01), "设备"="", "日志信息"="", "流程参数"=""} ("data in"), "时间标识"=w219, "设备"=w218, "日志信息"=w213) -> (w217:T17)
        n142 = call "氨氮操作日志.vi"("data in"=w217) -> ()  [unwired: 11 in]
      }
    }
    n143 = case shown="真" w142 {
      tunnel: w140 -> [_ w194]
      tunnel: w141 -> [_ w193]
      frame False {
      }
      frame True {
        n144 = case shown="\"水样测试\"" w193 {
          tunnel: [_ "【水样测试】" ("字符串") "【标样核查】" ("字符串") "【零点核查】" ("字符串") "【跨度核查】" ("字符串") "【空白测试】" ("字符串") "【平行样测试】" ("字符串") "【加标回收】" ("字符串") "【空白校准】" ("字符串") "【标样校准】" ("字符串")] -> w192
          frame "空闲", Default {
          }
          frame "水样测试" {
          }
          frame "标样核查" {
          }
          frame "零点核查" {
          }
          frame "跨度核查" {
          }
          frame "空白测试" {
          }
          frame "平行样测试" {
          }
          frame "加标回收" {
          }
          frame "空白校准" {
          }
          frame "标样校准" {
          }
        }
        n145 = case shown="1, 131" w194 {
          tunnel: [_ "总磷" ("table输入") "氨氮" ("table输入") "总氮" ("table输入")] -> w196
          frame Default {
          }
          frame 1, 131 {
          }
          frame 3, 92 {
          }
          frame 2, 76 {
          }
        }
        n146 = Concatenate Strings("-->>" ("字符串"), w192, "停止" ("字符串")) -> (w191:string)
        n147 = Get Date/Time In Seconds() -> (seconds since 1Jan1904=w197:timestamp)
        n148 = Bundle By Name(cluster=T17 {"时间标识"=timestamp(0 s since 1904-01-01), "设备"="", "日志信息"="", "流程参数"=""} ("data in"), "时间标识"=w197, "设备"=w196, "日志信息"=w191) -> (w195:T17)
        n149 = call "氨氮操作日志.vi"("data in"=w195) -> ()  [unwired: 11 in]
      }
    }
    n150 = case shown="1, 默认" w161 {
      selector: w161 -> [_ w301]
      tunnel: w164 -> [_ w302]
      tunnel: w163 -> [_ w300]
      frame 0 {
      }
      frame 1, Default {
        n151 = case shown="真" w300 {
          tunnel: w302 -> [_ w309]
          tunnel: w301 -> [_ w304]
          frame False {
          }
          frame True {
            n152 = case shown="默认" w304 {
              selector: w304 -> [w311 _ _ _ _ _]
              tunnel: [w310 "无故障" "电机故障" "温度故障" "通讯故障" "滴定故障"] -> w303
              frame Default {
                n153 = Format Into String(format string="%d" ("格式字符串"), initial string="内部故障-" ("工作状态"), w311) -> (resulting string=w310:string)  [unwired: 1 in, 1 out]
              }
              frame 0 {
              }
              frame 1 {
              }
              frame 2 {
              }
              frame 3 {
              }
              frame 4 {
              }
            }
            n154 = case shown="默认" w309 {
              tunnel: [_ "总磷" ("table输入") "氨氮" ("table输入") "总氮" ("table输入")] -> w305
              frame Default {
              }
              frame 1, 131 {
              }
              frame 3, 92 {
              }
              frame 2, 76 {
              }
            }
            n155 = Get Date/Time In Seconds() -> (seconds since 1Jan1904=w306:timestamp)
            n156 = Bundle By Name(cluster=T18 {"时间标识"=timestamp(0 s since 1904-01-01), "设备"="", "日志信息"=""} ("data in"), "时间标识"=w306, "设备"=w305, "日志信息"=w303) -> (w307:T18)
            n157 = call "氨氮报警信息.vi"("data in"=w307) -> ()  [unwired: 10 in, 1 out]
          }
        }
      }
    }
    n158 = case shown="真" w156 {
      frame False {
      }
      frame True {
        n159 = property on="多列列表框" class="MCListbox (严格)"() -> ("ItemNames"=w236:string[][], "Value"=w237:i32)  [unwired: 2 in, 2 out]
        n160 = Index Array(array=w236, index (row)=w237) -> (element=w235:string[])  [unwired: 1 in]
        n161 = Index Array(array=w235) -> (element=w234:string)  [unwired: 1 in]
        n162 = case shown="\"初始化\", \"读空白\", \"读取比色值\", \"读取空白值\", \"读数\", \"关阀\", \"关恒温\", \"加热消解\", \"降温\", \"结束\", \"进水样\", \"清洗\", \"清洗1\", \"润洗\", \"显色\", \"消解\", \"预热\", \"注入水样\"" w234 {
          selector: w234 -> [_ w240]
          frame Default {
          }
          frame "初始化", "读空白", "读取比色值", "读取空白值", "读数", "关阀", "关恒温", "加热消解", "降温", "结束", "进水样", "清洗", "清洗1", "润洗", "显色", "消解", "预热", "注入水样" {
            n163 = case shown="默认" w240 {
              selector: w240 -> [w244 w246]
              tunnel: [w244 w246] -> w239
              tunnel: [string[] [] ("数组") "数组"] -> w238
              frame "读数" {
              }
              frame Default {
              }
            }
            n164 = for {
              N: 1 -> [_]
              tunnel: w239 -> [w248]
              shift-right: [w247] -> w241
              shift-left: w238 -> [w249]
              n165 = Search 1D Array(1D array=w249, element=w248) -> (index of element=w252:i32)  [unwired: 1 in]
              n166 = Format Into String(format string="%s" ("格式字符串"), w248) -> (resulting string=w253:string)  [unwired: 2 in, 1 out]
              n167 = Equal?(x=w252, y=-1) -> (x = y?=w250:bool)
              n168 = case shown="真" w250 {
                tunnel: w253 -> [_ w261]
                tunnel: w249 -> [w255 w265]
                tunnel: w248 -> [_ w264]
                tunnel: [w255 w263] -> w247
                frame False {
                }
                frame True {
                  n169 = Insert Into Array(array=w265, new element=w264) -> (w263:string[])  [unwired: 1 in]
                  n170 = case shown="\"结束\"" w261 {
                    selector: w261 -> [w290 w293 w296]
                    tunnel: [w290 w292 w295] -> w257
                    frame Default {
                    }
                    frame "初始化" {
                      n171 = Concatenate Strings("-->>" ("字符串"), w293) -> (w292:string)
                    }
                    frame "结束" {
                      n172 = Concatenate Strings("-->>" ("字符串"), w296) -> (w295:string)
                    }
                  }
                  n173 = global read "VAR氨氮全局变量.vi" "状态告警区"() -> (w260:T5)
                  n174 = Unbundle By Name(w260) -> ("工作状态"=w259:T9)
                  n175 = global read "VAR氨氮全局变量.vi" "状态告警区"() -> (w280:T5)
                  n176 = case shown="\"水样测试\"" w259 {
                    tunnel: [_ "【水样测试】" ("字符串") "【标样核查】" ("字符串") "【零点核查】" ("字符串") "【跨度核查】" ("字符串") "【空白测试】" ("字符串") "【平行样测试】" ("字符串") "【加标回收】" ("字符串") "【空白校准】" ("字符串") "【标样校准】" ("字符串")] -> w258
                    frame "空闲", Default {
                    }
                    frame "水样测试" {
                    }
                    frame "标样核查" {
                    }
                    frame "零点核查" {
                    }
                    frame "跨度核查" {
                    }
                    frame "空白测试" {
                    }
                    frame "平行样测试" {
                    }
                    frame "加标回收" {
                    }
                    frame "空白校准" {
                    }
                    frame "标样校准" {
                    }
                  }
                  n177 = Unbundle By Name(w280) -> ("id"=w279:u16)
                  n178 = global read "VAR氨氮全局变量.vi" "状态告警区"() -> (w275:T5)
                  n179 = case shown="1, 131" w279 {
                    tunnel: [_ "总磷" ("table输入") "氨氮" ("table输入") "总氮" ("table输入")] -> w277
                    frame Default {
                    }
                    frame 1, 131 {
                    }
                    frame 3, 92 {
                    }
                    frame 2, 76 {
                    }
                  }
                  n180 = Unbundle By Name(w275) -> ("F0"=w272:sgl, "F1"=w271:sgl, "F2"=w270:sgl, "F3"=w269:sgl, "id"=w268:u16, "flowid"=w267:u16, "量程"=w266:u16)
                  n181 = Concatenate Strings(w258, w257) -> (w256:string)
                  n182 = Format Into String(format string="F0=%#f,F1=%#f,F2=%#f,F3=%#f,Flow=%d-%-d-%-d" ("格式字符串"), w272, w271, w270, w269, w268, w267, w266) -> (resulting string=w273:string)  [unwired: 2 in, 1 out]
                  n183 = Get Date/Time In Seconds() -> (seconds since 1Jan1904=w276:timestamp)
                  n184 = Bundle By Name(cluster=T17 {"时间标识"=timestamp(0 s since 1904-01-01), "设备"="", "日志信息"="", "流程参数"=""} ("data in"), "时间标识"=w276, "设备"=w277, "日志信息"=w256, "流程参数"=w273) -> (w278:T17)
                  n185 = call "氨氮操作日志.vi"("data in"=w278) -> ()  [unwired: 11 in]
                }
              }
            }
            n186 = local write "数组"(w241) -> ()
          }
        }
      }
    }
    n187 = call <vilib>:"Boolean Crossing PtByPt.vi"("input"=w183) -> ("crossing"=w147:bool)  [unwired: 2 in]
    n188 = Bundle By Name(cluster=T16 {"启动模式"=enum."跨度核查", "启动参数"=1, "量程"=enum."低量程"} ("参数簇"), "启动参数"=w178, "启动模式"=w180, "量程"=w179) -> (w172:T16)
    n189 = First Call?() -> (First Call?: T/F=w184:bool)
    n190 = Or(x=w147, y=w184) -> (x .or. y?=w182:bool)
    n191 = while {
      tunnel: w182 -> [w382]
      tunnel: w172 -> [w381]
      shift-right: [w376] -> _
      shift-left: _ -> [w378]
      shift-right: [w377] -> _
      shift-left: _ -> [w379]
      stop <- TRUE stop-if-true
      n192 = case shown="真" w382 {
        tunnel: [w384 w392] -> w377
        tunnel: [w383 w391] -> w376
        tunnel: w381 -> [_ w386]
        tunnel: w379 -> [w384 _]
        tunnel: w378 -> [w383 _]
        frame False {
        }
        frame True {
          n193 = call "斯坦道XML解析.vi"("添加的路径"="流程路径", "参数簇"=w386) -> ("步骤时间"=w387:string[], "步骤名"=w389:string[])  [unwired: 8 in]
          n194 = for {
            tunnel: w389 -> [_] mode=indexing
            tunnel: [w393] -> w390 mode=indexing
            i -> [w393]
          }
          n195 = Build Array(w389, w387) -> (w388:string[][])
          n196 = Transpose 2D Array(2D array=w388) -> (transposed array=w391:string[][])
          n197 = Number To Decimal String(number=w390) -> (decimal integer string=w392:string[])  [unwired: 1 in]
        }
      }
      n198 = property on="多列列表框" class="MCListbox (严格)"("ItemNames"=w376, "RowHdrs[]"=w377) -> ()  [unwired: 2 in, 2 out]
    }
    n199 = case shown="1, 默认" w166 {
      selector: w166 -> [_ w323]
      tunnel: w169 -> [_ w324]
      tunnel: w168 -> [_ w322]
      frame 0 {
      }
      frame 1, Default {
        n200 = case shown="真" w322 {
          tunnel: w324 -> [_ w331]
          tunnel: w323 -> [_ w325]
          frame False {
          }
          frame True {
            n201 = case shown="默认" w325 {
              selector: w325 -> [w333 _ _ _ _ _ _ _ _ _ _ _ _ _ _ _ _ _ _ _ _ _ _ _ _ _ _ _ _ _ _ _ _ _ _ _ _ _]
              tunnel: [w332 "无告警" "缺试剂告警" "缺水样告警" "缺蒸馏水告警" "缺标液告警" "仪表漏液告警" "标定异常告警" "超量程告警" "加热异常" "低试剂预警" "超上限告警" "超下限告警" "仪表内部其他异常" "滴定异常告警" "电极异常告警" "量程切换告警" "参数设置告警" "PH电极电位异常" "电导率电极异常" "浊度光度异常" "溶解氧电极异常" "溶解氧光强异常" "温度异常告警" "PH异常告警" "溶解氧异常告警" "电导率异常告警" "浊度异常告警" "叶绿素异常告警" "藻密度异常告警" "蓝绿藻异常告警" "ORP异常告警" "氨氮异常告警" "清洁刷异常告警" "SD卡异常告警" "蓝牙异常告警" "WiFi异常告警" "流程异常告警"] -> w326
              frame Default {
                n202 = Format Into String(format string="%d" ("格式字符串"), initial string="内部告警-" ("工作状态"), w333) -> (resulting string=w332:string)  [unwired: 1 in, 1 out]
              }
              frame 0 {
              }
              frame 1 {
              }
              frame 2 {
              }
              frame 3 {
              }
              frame 4 {
              }
              frame 5 {
              }
              frame 6 {
              }
              frame 7 {
              }
              frame 8 {
              }
              frame 9 {
              }
              frame 10 {
              }
              frame 11 {
              }
              frame 12 {
              }
              frame 13 {
              }
              frame 14 {
              }
              frame 15 {
              }
              frame 16 {
              }
              frame 17 {
              }
              frame 18 {
              }
              frame 19 {
              }
              frame 20 {
              }
              frame 21 {
              }
              frame 22 {
              }
              frame 23 {
              }
              frame 24 {
              }
              frame 25 {
              }
              frame 26 {
              }
              frame 27 {
              }
              frame 28 {
              }
              frame 29 {
              }
              frame 30 {
              }
              frame 31 {
              }
              frame 32 {
              }
              frame 33 {
              }
              frame 34 {
              }
              frame 35 {
              }
              frame 36 {
              }
            }
            n203 = case shown="3, 92" w331 {
              tunnel: ["总磷" ("table输入") "氨氮" ("table输入") "总氮" ("table输入")] -> w327
              frame 1, 131 {
              }
              frame 3, 92 {
              }
              frame 2, 76, Default {
              }
            }
            n204 = Get Date/Time In Seconds() -> (seconds since 1Jan1904=w328:timestamp)
            n205 = Bundle By Name(cluster=T18 {"时间标识"=timestamp(0 s since 1904-01-01), "设备"="", "日志信息"=""} ("data in"), "时间标识"=w328, "设备"=w327, "日志信息"=w326) -> (w329:T18)
            n206 = call "氨氮报警信息.vi"("data in"=w329) -> ()  [unwired: 10 in, 1 out]
          }
        }
      }
    }
  }
  n207 = while {
    tunnel: w13 -> [w409]
    tunnel: [w407] -> _
    stop <- FALSE stop-if-true
    # "定时更新"
    n208 = Get Queue Status(queue=w409) -> (queue out=w406:refnum<queue>, # elements in queue=w405:i32)  [unwired: 2 in, 6 out]
    n209 = case shown="0" w405 {
      tunnel: [_ w412] -> w407
      tunnel: w406 -> [_ w411]
      frame Default {
      }
      frame 0 {
        w415 = u16 3 items=["总磷"=1, "氨氮"=3] ("站号")
        n210 = call "版本号读取.vi"() -> ("error out"=w412:errorcluster, "固件版本号"=→"固件版本号":string)  [unwired: 10 in]
        n211 = Bundle By Name(cluster=cluster{"命令":string, "data":variant} {"命令"="", "data"=variant} ("元素"), "命令"="读序列号", "data"=w415) -> (w414:cluster{"命令":string, "data":variant})
        n212 = Enqueue Element(queue=w411, element=w414) -> ()  [unwired: 2 in, 3 out]
      }
    }
    n213 = Wait (ms)(milliseconds to wait=u32 1000 ("等待时间（毫秒）")) -> ()  [unwired: 1 out]
  }
  n214 = Bundle("参数下拉列表"=w5, "测量模式下拉列表"=w4, "量程下拉列表"=w3) -> (w6:T20)  [unwired: 1 in]
  n215 = Obtain Notifier(name (unnamed)="NH3N" ("名称（未命名）"), notification data type=FALSE) -> (notifier out=w9:refnum<notifier>)  [unwired: 2 in, 2 out]
  n216 = property on="曲线模型" class="曲线模型 (严格)"("属性"=w6) -> (error out=w12:errorcluster)  [unwired: 2 in, 1 out]
  n217 = Cancel Notification(0:w9) -> (8:w8:refnum<notifier>)  [unwired: 1 in, 2 out]
  n218 = Obtain Queue(name (unnamed)="NH3N" ("名称（未命名）"), element data type=cluster{"命令":string, "data":variant} {"命令"="", "data"=variant}) -> (queue out=w21:refnum<queue>, error out=w22:errorcluster)  [unwired: 3 in, 1 out]
  n219 = while {
    tunnel: w21 -> [w423]
    tunnel: w22 -> [_]
    stop <- FALSE stop-if-true
    n220 = Get Queue Status(queue=w423) -> (queue out=w419:refnum<queue>, # elements in queue=w418:i32)  [unwired: 2 in, 6 out]
    n221 = Wait (ms)(milliseconds to wait=u32 1000 ("等待时间（毫秒）")) -> ()  [unwired: 1 out]
    n222 = global read "氨氮断电保存全局变量.vi" "流程路径"() -> (w422:path)
    n223 = case shown="0" w418 {
      tunnel: w419 -> [_ w426]
      frame Default {
      }
      frame 0 {
        w435 = u16 3 items=["总磷"=1, "氨氮"=3] ("站号")
        # "试剂填充 172 \n管路清洗108\n氨氮92\n总磷131\n总磷海水147\n总氮76\n总氮海水92"
        n224 = global read "VAR氨氮全局变量.vi" "状态告警区"() -> (w427:T5)
        n225 = Bundle By Name(cluster=cluster{"命令":string, "data":variant} {"命令"="", "data"=variant} ("元素"), "命令"="读状态告警区", "data"=w435) -> (w441:cluster{"命令":string, "data":variant})
        n226 = Bundle By Name(cluster=cluster{"命令":string, "data":variant} {"命令"="", "data"=variant} ("元素"), "命令"="读测量数据区", "data"=w435) -> (w438:cluster{"命令":string, "data":variant})
        n227 = Unbundle By Name(w427) -> ("系统时间"=w434:timestamp)
        n228 = Enqueue Element(queue=w426, element=w441) -> (queue out=w436:refnum<queue>)  [unwired: 2 in, 2 out]
        n229 = Get Date/Time In Seconds() -> (seconds since 1Jan1904=w433:timestamp)
        n230 = Subtract(x=w433, y=w434) -> (x-y=w432:dbl)
        n231 = Absolute Value(x=w432) -> (abs(x)=w431:dbl)
        n232 = Enqueue Element(queue=w436, element=w438) -> (queue out=w428:refnum<queue>)  [unwired: 2 in, 2 out]
        n233 = Greater Or Equal?(x=w431, y=120.0) -> (x >= y?=w429:bool)
        n234 = case shown="真" w429 {
          tunnel: w428 -> [_ w444]
          frame False {
          }
          frame True {
            n235 = call "氨氮启动命令.vi"("参数"=T21 {"站号"=3, "量程切换"=enum."AUTO", "控制命令"=enum."校时", "模式设置"=enum."待机", "测量间隔"=0}) -> ("启动命令"=w443:cluster{"命令":string, "data":variant})  [unwired: 10 in]
            n236 = Enqueue Element(queue=w444, element=w443) -> ()  [unwired: 2 in, 3 out]
          }
        }
      }
    }
    n237 = local write "流程路径"(w422) -> ()
    n238 = global read "氨氮断电保存全局变量.vi" "MB通信方式选择"() -> (w420:enum16{"串口", "TCP"})
    n239 = case shown="\"TCP\"" w420 {
      tunnel: [w446 w447] -> w421
      frame "串口", Default {
        n240 = global read "氨氮断电保存全局变量.vi" "VISA Resource"() -> (w446:refnum<visa-resource-name>)
      }
      frame "TCP" {
        n241 = global read "氨氮断电保存全局变量.vi" "IP"() -> (w447:string)
      }
    }
    "字符串" <- w421
  }
  n242 = control-ref of="测量模式下拉列表"() -> (w18:refnum<vi>)
  n243 = control-ref of="量程参数读取"() -> (w7:refnum<vi>)
  n244 = control-ref of="参数下拉列表"() -> (w19:refnum<vi>)
  n245 = control-ref of="量程下拉列表"() -> (w20:refnum<vi>)
  n246 = control-ref of="公式"() -> (w17:refnum<vi>)
  n247 = while {
    tunnel: w21 -> [w454]
    tunnel: w20 -> [w453]
    tunnel: w19 -> [w452]
    tunnel: w18 -> [w451]
    tunnel: w17 -> [w450]
    tunnel: w7 -> [w449]
    tunnel: w12 -> [_]
    tunnel: w8 -> [w448]
    stop <- FALSE stop-if-true
    n248 = event shown="[13] \"单步测试\": 值改变" {
      selector: _ -> [_ _ _ _ _ _ _ _ _ _ _ _ _ _ _ _ _ _ _ _ _ _]
      dyn-events: _ -> [_ _ _ _ _ _ _ _ _ _ _ _ _ _ _ _ _ _ _ _ _ _]
      timeout: _ -> [_ _ _ _ _ _ _ _ _ _ _ _ _ _ _ _ _ _ _ _ _ _]
      tunnel: w454 -> [_ _ _ _ w474 w488 _ _ _ _ _ _ w534 w543 w550 _ _ _ _ _ _ _]
      tunnel: w453 -> [_ _ _ _ _ _ _ _ _ _ _ _ _ _ _ _ _ _ w566 _ _ _]
      tunnel: w452 -> [_ _ _ _ _ _ _ _ _ _ _ _ _ _ _ _ _ _ w564 _ w582 w589]
      tunnel: w451 -> [_ _ _ _ _ _ _ _ _ _ _ _ _ _ _ _ _ _ w565 _ _ _]
      tunnel: w450 -> [_ _ _ _ _ _ _ _ _ _ _ _ _ _ _ _ _ _ w560 _ _ _]
      tunnel: w449 -> [_ _ _ _ _ _ _ _ _ _ _ _ _ _ _ _ _ _ _ _ w580 _]
      tunnel: w448 -> [_ _ _ _ _ _ _ _ _ _ _ _ _ _ w545 _ _ _ _ _ _ _]
      tunnel: [_ _ _ w460 _ _ _ _ _ _ _ _ _ _ _ _ _ _ _ _ _ _] -> _
      event Timeout {
        n249 = event-data() -> ()  [unwired: 1 in, 3 out]
      }
      event "布尔": Mouse Down {
        n250 = event-data() -> ("CtlRef"=w457:refnum<vi>)  [unwired: 1 in, 5 out]
        n251 = property class="Bool (严格)"(reference=w457) -> ("Value"=w456:bool)  [unwired: 1 in, 2 out]
        n252 = case shown="真" w456 {
          frame False {
            n253 = call "密码键盘.vi"() -> ("NewNumber"=→"输入密码":dbl)  [unwired: 1 in]
          }
          frame True {
            n254 = local write "输入密码"(u32 0 ("输入密码")) -> ()
          }
        }
      }
      event "流程固件": Value Change {
        n255 = event-data() -> ()  [unwired: 1 in, 6 out]
        n256 = call "流程固件设置对话框.vi"() -> ()  [unwired: 12 in]
      }
      event "测量模式下拉列表", "量程下拉列表", "参数下拉列表": Value Change {
        n257 = event-data() -> ()  [unwired: 1 in, 6 out]
        n258 = local read "测量模式下拉列表"() -> (w463:enum16{"水样测量", "零点核查", "跨度核查", "标样核查", "加标回收"})
        n259 = local read "参数下拉列表"() -> (w462:enum16{"总磷", "总氮", "氨氮"})
        n260 = local read "量程下拉列表"() -> (w464:enum16{"低量程", "高量程"})
        n261 = Bundle("参数下拉列表"=w462, "测量模式下拉列表"=w463, "量程下拉列表"=w464) -> (w461:T20)  [unwired: 1 in]
        n262 = property on="曲线模型" class="曲线模型 (严格)"("属性"=w461) -> (error out=w460:errorcluster)  [unwired: 2 in, 1 out]
      }
      event "串口设置": Value Change {
        n263 = event-data() -> ()  [unwired: 1 in, 6 out]
        n264 = global read "氨氮断电保存全局变量.vi" "MB通信方式选择"() -> (w465:enum16{"串口", "TCP"})
        n265 = global read "氨氮断电保存全局变量.vi" "VISA Resource"() -> (w471:refnum<visa-resource-name>)
        n266 = global read "氨氮断电保存全局变量.vi" "PORT"() -> (w469:string)
        n267 = global read "氨氮断电保存全局变量.vi" "IP"() -> (w470:string)
        n268 = call "串口配置.vi"("PORT"=w469, "IP"=w470, "MB通信方式选择"=w465, "请选择串口:"=w471) -> ("PORT 2"=w467:string, "IP 2"=w468:string, "确认 2"=w472:bool, "VISA资源名称 2"=w473:refnum<visa-resource-name>, "MB通信方式选择 2"=w466:enum16{"串口", "TCP"})  [unwired: 3 in]
        n269 = case shown="真" w472 {
          tunnel: w473 -> [_ w479]
          tunnel: w474 -> [_ w478]
          tunnel: w468 -> [_ w477]
          tunnel: w467 -> [_ w476]
          tunnel: w466 -> [_ w475]
          frame False {
          }
          frame True {
            n270 = flat-sequence {
              tunnel: w479 -> [w484]
              tunnel: w478 -> [w485]
              tunnel: w477 -> [w483]
              tunnel: w476 -> [w482]
              tunnel: w475 -> [w481]
              frame #0 {
                n271 = global write "氨氮断电保存全局变量.vi" "IP"(w483) -> ()
                n272 = global write "氨氮断电保存全局变量.vi" "PORT"(w482) -> ()
                n273 = global write "氨氮断电保存全局变量.vi" "VISA Resource"(w484) -> ()
                n274 = global write "氨氮断电保存全局变量.vi" "MB通信方式选择"(w481) -> ()
                n275 = Flush Queue(queue=w485) -> (queue out=w480:refnum<queue>)  [unwired: 1 in, 2 out]
                n276 = Enqueue Element(queue=w480, element=cluster{"命令":string, "data":variant} {"命令"="启用模块", "data"=variant} ("元素")) -> ()  [unwired: 2 in, 3 out]
              }
              frame #1 {
                n277 = call "配置文件保存.vi"() -> ()  [unwired: 12 in]
              }
            }
          }
        }
      }
      event "模块启用": Value Change {
        n278 = event-data() -> ("OldVal"=w489:bool)  [unwired: 1 in, 5 out]
        n279 = Flush Queue(queue=w488) -> (queue out=w487:refnum<queue>)  [unwired: 1 in, 2 out]
        n280 = case shown="假" w489 {
          tunnel: w487 -> [w490 w492]
          frame False {
            n281 = Enqueue Element(queue=w490, element=cluster{"命令":string, "data":variant} {"命令"="停用模块", "data"=variant} ("元素")) -> ()  [unwired: 2 in, 3 out]
          }
          frame True {
            n282 = Enqueue Element(queue=w492, element=cluster{"命令":string, "data":variant} {"命令"="启用模块", "data"=variant} ("元素")) -> ()  [unwired: 2 in, 3 out]
          }
        }
      }
      event "流程路径": Value Change {
        n283 = event-data() -> ()  [unwired: 1 in, 6 out]
        n284 = flat-sequence {
          frame #0 {
            n285 = local read "流程路径"() -> (w494:path)
            n286 = global write "氨氮断电保存全局变量.vi" "流程路径"(w494) -> ()
          }
          frame #1 {
            n287 = call "配置文件保存.vi"() -> ()  [unwired: 12 in]
          }
        }
      }
      event "公式一键写入": Value Change {
        n288 = event-data() -> ()  [unwired: 1 in, 6 out]
        n289 = local read "公式"() -> (w495:cluster{"X^2":dbl, "X":dbl, "b":dbl})
        n290 = call "公式复合写入.vi"("公式"=w495) -> ()  [unwired: 11 in]
      }
      event "曲线模型": Value Change {
        n291 = event-data() -> ()  [unwired: 1 in, 6 out]
        n292 = local write "公式"("曲线模型") -> ()
      }
      event "质控参数设置": Value Change {
        n293 = event-data() -> ()  [unwired: 1 in, 6 out]
        n294 = global read "氨氮断电保存全局变量.vi" "质控参数设置"() -> (w497:T22)
        n295 = call "质控参数设置.vi"("质控参数设置"=w497) -> ("输出簇"=w498:T23)  [unwired: 10 in]
        n296 = Unbundle By Name(w498) -> ("确定"=w499:bool)
        n297 = case shown="真" w499 {
          tunnel: w498 -> [_ w501]
          tunnel: w497 -> [_ w500]
          frame False {
          }
          frame True {
            n298 = flat-sequence {
              tunnel: w501 -> [w508]
              tunnel: w500 -> [w507]
              frame #0 {
                n299 = Unbundle By Name(w508) -> ("跨度值"=w506:dbl, "零点标准液浓度"=w505:dbl, "跨度标准液浓度"=w504:dbl, "标准液标准浓度"=w503:dbl)
                n300 = Bundle By Name(cluster=w507, "跨度值"=w506, "零点标准液浓度"=w505, "跨度标准液浓度"=w504, "标准液标准浓度"=w503) -> (w502:T22)
                n301 = global write "氨氮断电保存全局变量.vi" "质控参数设置"(w502) -> ()
              }
              frame #1 {
                n302 = call "配置文件保存.vi"() -> ()  [unwired: 12 in]
              }
            }
          }
        }
      }
      event "仪器参数设置": Value Change {
        n303 = event-data() -> ()  [unwired: 1 in, 6 out]
        n304 = global read "氨氮断电保存全局变量.vi" "氨氮仪器参数"() -> (w509:T24)
        n305 = call "仪器参数设置.vi"("仪器参数设置"=w509) -> ("仪器参数设置输出"=w510:T25)  [unwired: 10 in]
        n306 = Unbundle By Name(w510) -> ("确定"=w511:bool)
        n307 = case shown="真" w511 {
          tunnel: w510 -> [_ w513]
          tunnel: w509 -> [_ w512]
          frame False {
          }
          frame True {
            n308 = flat-sequence {
              tunnel: w513 -> [w530]
              tunnel: w512 -> [w529]
              frame #0 {
                n309 = Unbundle By Name(w530) -> ("测量量程"=w528:dbl, "测量精度"=w527:dbl, "测量间隔"=w526:dbl, "消解温度"=w525:dbl, "消解时长"=w523:dbl, "空白校准时间"=w522:timestamp, "曲线截距"=w521:dbl, "曲线斜率"=w520:dbl, "测量检出限"=w519:dbl, "测量信号值"=w518:dbl, "线性相关系数"=w517:dbl, "二次多项式系数"=w516:dbl, "标样校准时间"=w515:timestamp, "单位"=w514:u16)
                n310 = Bundle By Name(cluster=w529, "测量量程"=w528, "测量精度"=w527, "测量间隔"=w526, "消解温度"=w525, "消解时长"=w523, "空白校准时间"=w522, "曲线截距"=w521, "曲线斜率"=w520, "测量检出限"=w519, "测量信号值"=w518, "线性相关系数"=w517, "二次多项式系数"=w516, "标样校准时间"=w515, "单位"=w514) -> (w524:T24)
                n311 = global write "氨氮断电保存全局变量.vi" "氨氮仪器参数"(w524) -> ()
              }
              frame #1 {
                n312 = call "配置文件保存.vi"() -> ()  [unwired: 12 in]
              }
            }
          }
        }
      }
      event "自动测试量程配置": Value Change {
        n313 = event-data() -> ()  [unwired: 1 in, 6 out]
        n314 = flat-sequence {
          frame #0 {
            n315 = global write "氨氮断电保存全局变量.vi" "自动测试量程配置"("自动测试量程配置") -> ()
          }
          frame #1 {
            n316 = call "配置文件保存.vi"() -> ()  [unwired: 12 in]
          }
        }
      }
      event "手动启动": Value Change {
        n317 = event-data() -> ()  [unwired: 1 in, 6 out]
        n318 = call "氨氮启动参数对话框.vi"() -> ("确认"=w532:bool, "元素"=w533:cluster{"命令":string, "data":variant})  [unwired: 10 in]
        n319 = case shown="真" w532 {
          tunnel: w534 -> [_ w536]
          tunnel: w533 -> [_ w535]
          frame False {
          }
          frame True {
            n320 = Enqueue Element(queue=w536, element=w535) -> ()  [unwired: 2 in, 3 out]
          }
        }
      }
      event "单步测试": Value Change {
        w538 = u16 1 items=["总磷"=1, "氨氮"=3] ("站号")
        n321 = event-data() -> ()  [unwired: 1 in, 6 out]
        n322 = Bundle("站号"=w538, "总磷氨氮调试"="总磷氨氮调试") -> (w537:cluster{"站号":u16, "总磷氨氮调试":u16[]})  [unwired: 1 in]
        n323 = Bundle By Name(cluster=cluster{"命令":string, "data":variant} {"命令"="", "data"=variant} ("元素"), "命令"="debug", "data"=w537) -> (w540:cluster{"命令":string, "data":variant})
        n324 = Enqueue Element(queue=w543, element=w540) -> ()  [unwired: 2 in, 3 out]
      }
      event "停止": Value Change {
        n325 = event-data() -> ()  [unwired: 1 in, 6 out]
        n326 = Enqueue Element(queue=w550, element=cluster{"命令":string, "data":variant} {"命令"="启动", "data"=variant(cluster{"站号":u16, "控制命令输出":u16[]} {"站号"=1, "控制命令输出"=[2816]})} ("元素")) -> (queue out=w547:refnum<queue>)  [unwired: 2 in, 2 out]
        n327 = Cancel Notification(0:w545) -> (8:w546:refnum<notifier>)  [unwired: 1 in, 2 out]
        n328 = Send Notification(notification=TRUE ("通知"), notifier=w546) -> ()  [unwired: 1 in, 2 out]
        n329 = Enqueue Element(queue=w547, element=cluster{"命令":string, "data":variant} {"命令"="启动", "data"=variant(cluster{"站号":u16, "控制命令输出":u16[]} {"站号"=2, "控制命令输出"=[2816]})} ("元素")) -> ()  [unwired: 2 in, 3 out]
      }
      event "设置": Value Change {
        n330 = event-data() -> ()  [unwired: 1 in, 6 out]
        n331 = property on="窗格" class="Pane"("Origin"=T7 {"Horizontal"=0, "Vertical"=628} ("原点")) -> ()  [unwired: 2 in, 2 out]
      }
      event "返回": Value Change {
        n332 = event-data() -> ()  [unwired: 1 in, 6 out]
        n333 = property on="窗格" class="Pane"("Origin"=T7 {"Horizontal"=0, "Vertical"=0} ("原点")) -> ()  [unwired: 2 in, 2 out]
      }
      event "公式.X^2", "公式.X", "公式.b": Mouse Down {
        n334 = event-data() -> ("CtlRef"=w556:refnum<vi>)  [unwired: 1 in, 5 out]
        n335 = property class="DigNum (严格)"(reference=w556) -> (reference out=w554:refnum<vi>, "Value"=w555:dbl)  [unwired: 1 in, 1 out]
        n336 = call "数字键盘.vi"("OldNumber"=w555) -> ("NewNumber"=w553:dbl)
        n337 = property class="DigNum (严格)"(reference=w554, "Val(Sgnl)"=w553) -> ()  [unwired: 1 in, 2 out]
      }
      event "读公式": Value Change {
        n338 = event-data() -> ()  [unwired: 1 in, 6 out]
        n339 = property class="Enum (严格)"(reference=w565) -> ("Value"=w562:enum16{"水样测量", "零点核查", "跨度核查", "标样核查", "加标回收"})  [unwired: 1 in, 2 out]
        n340 = property class="Enum (严格)"(reference=w564) -> ("Value"=w563:enum16{"总磷", "总氮", "氨氮"})  [unwired: 1 in, 2 out]
        n341 = property class="Enum (严格)"(reference=w566) -> ("Value"=w561:enum16{"低量程", "高量程"})  [unwired: 1 in, 2 out]
        n342 = call "公式读取.vi"("量程"=w561, "测量模式"=w562, "测量参数"=w563) -> ("error out"=w558:errorcluster, "公式"=w559:cluster{"X^2":dbl, "X":dbl, "b":dbl})  [unwired: 7 in]
        n343 = property class="Clust (严格)"(reference=w560, "Value"=w559) -> ()  [unwired: 1 in, 2 out]
        n344 = case shown="错误" w558 {
          tunnel: ["读取成功" ("消息") "读取失败" ("消息")] -> w557
          frame No Error {
          }
          frame Error {
          }
        }
        n345 = One Button Dialog(message=w557) -> ()  [unwired: 1 in, 1 out]
      }
      event "写公式": Value Change {
        n346 = event-data() -> ()  [unwired: 1 in, 6 out]
        n347 = call "公式写入.vi"("公式"="公式", "量程"="量程下拉列表", "测量模式"="测量模式下拉列表", "测量参数"="参数下拉列表") -> ("error out"=w571:errorcluster)  [unwired: 7 in]
        n348 = case shown="无错误" w571 {
          tunnel: ["写入成功" ("消息") "写入失败" ("消息")] -> w572
          frame No Error {
          }
          frame Error {
          }
        }
        n349 = One Button Dialog(message=w572) -> ()  [unwired: 1 in, 1 out]
      }
      event "量程切换阈值读取": Value Change {
        n350 = event-data() -> ()  [unwired: 1 in, 6 out]
        n351 = property class="Enum (严格)"(reference=w582) -> ("Value"=w581:enum16{"总磷", "总氮", "氨氮"})  [unwired: 1 in, 2 out]
        n352 = call "量程读取.vi"("测量参数"=w581) -> ("error out"=w577:errorcluster, "量程参数读取"=w579:T26)  [unwired: 9 in]
        n353 = property class="Clust (严格)"(reference=w580, "Value"=w579) -> ()  [unwired: 1 in, 2 out]
        n354 = case shown="错误" w577 {
          tunnel: ["读取成功" ("消息") "读取失败" ("消息")] -> w578
          frame No Error {
          }
          frame Error {
          }
        }
        n355 = One Button Dialog(message=w578) -> ()  [unwired: 1 in, 1 out]
      }
      event "量程切换阈值写入": Value Change {
        n356 = event-data() -> ()  [unwired: 1 in, 6 out]
        n357 = property class="Enum (严格)"(reference=w589) -> ("Value"=w588:enum16{"总磷", "总氮", "氨氮"})  [unwired: 1 in, 2 out]
        n358 = call "量程写入.vi"("量程参数写入"="量程参数读取", "测量参数"=w588) -> ("error out"=w586:errorcluster)  [unwired: 8 in]
        n359 = case shown="无错误" w586 {
          tunnel: ["写入成功" ("消息") "写入失败" ("消息")] -> w587
          frame No Error {
          }
          frame Error {
          }
        }
        n360 = One Button Dialog(message=w587) -> ()  [unwired: 1 in, 1 out]
      }
    }
  }
  n361 = while {
    tunnel: [w599] -> _
    shift-right: [w597] -> _
    shift-left: _ -> [w596]
    tunnel: w1 -> [w593]
    stop <- FALSE stop-if-true
    n362 = global read "VAR氨氮全局变量.vi" "配置文件 path"() -> (w592:path)
    n363 = Wait (ms)(milliseconds to wait=u32 1000 ("等待时间（毫秒）")) -> ()  [unwired: 1 out]
    n364 = Get File Size(file=w592, error in=w593) -> (size (in bytes)=w597:i64, 0:w594:errorcluster)  [unwired: 1 out]
    n365 = Not Equal?(x=w597, y=w596) -> (x != y?=w595:bool)
    n366 = case shown="真" w595 {
      tunnel: [w601 w605] -> w599
      tunnel: w592 -> [_ w604]
      tunnel: w594 -> [w601 w603]
      frame False {
      }
      frame True {
        # "文件发生改变进行更新"
        n367 = vi-ref "氨氮断电保存全局变量.vi"() -> (w602:refnum<vi>)
        n368 = call <vilib>:"Open Config Data.vi"("error in (no error)"=w603, "configuration file path"=w604) -> ("error out"=w609:errorcluster, "refnum"=w608:T6)  [unwired: 7 in, 1 out]
        n369 = call <userlib>:"Read Panel from INI__ogtk.vi"("error in (no error)"=w609, "VI ref"=w602, "refnum"=w608) -> ("error out"=w607:errorcluster, "refnum out"=w606:T6)  [unwired: 7 in]
        n370 = call <vilib>:"Close Config Data.vi"("error in (no error)"=w607, "refnum"=w606) -> ("error out"=w605:errorcluster)  [unwired: 8 in, 1 out]
      }
    }
  }
